vi "HTTPRPC.vi"(6 "error in (no error)":errorcluster, 9 "Address":string) -> (0 "error out":errorcluster, 3 "mbed.lvclass":refnum<class "mbed.lvclass">)   [LabVIEW 2011, in "mbed_LVLibrary.lvlib" / "HTTPRPC.lvclass"]
uses:
  HTTPRPC.lvclass
  mbed/mbed.lvclass
  HTTPRPC.lvclass/HTTPRPC.ctl
panel:
  in  "mbed_LVLibrary.lvlib:HTTPRPC.lvclass":refnum<class "HTTPRPC.lvclass">
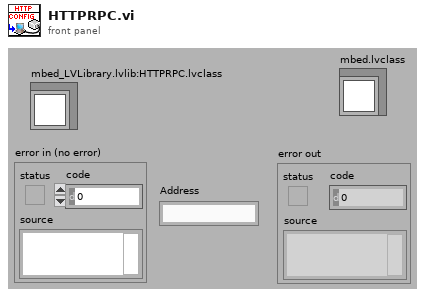
[diagram p1: front panel]
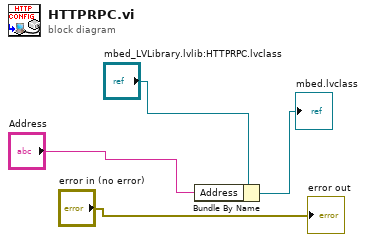
[diagram p0: block diagram]
diagram:
  n1 = Bundle By Name(cluster="mbed_LVLibrary.lvlib:HTTPRPC.lvclass", "Address"="Address") -> (→"mbed.lvclass":refnum<class "HTTPRPC.lvclass">)
  "error out" <- "error in (no error)"
